vi "canDataSort.vi"() -> ()   [LabVIEW 2023] (continued)
  68\t00\t97\tCC\t00\t16\t39\t67\r\n      1542  18F120F0   00000004    8        2B\t75\t60\tB1\tB0\t01\tFF\tFF\r\n      1563  0CF101A7   00000004    8        68\t00\t97\tCC\t00\t16\t39\t68\r\n      1562  1FFFFFFF   00000004    8        00\t00\tFF\tFF\tFF\tFF\tFF\tFF\r\n      1552  1FFFFFFF   00000004    8        00\t00\tFF\tFF\tFF\tFF\tFF\tFF\r\n      1547  1FFFFFFF   00000004    8        00\t00\tFF\tFF\tFF\tFF\tFF\tFF\r\n      1546  18F121F0   00000004    8        09\t18\t00\t00\tFF\tFF\tB0\t01\r\n      1545  18F106A7   00000004    8        00\tF7\tFF\tFF\tFF\tFF\tFF\t8F\r\n      1545  0CF104A7   00000004    8        F0\t60\t22\tFC\tFF\tFF\tFF\t47\r\n      1544  0CF103A7   00000004    8        17\t1F\t08\t60\tB1\t1F\t08\t47\r\n      1544  0CF102A7   00000004    8        30\t75\tE0\t2E\t80\tFF\tFF\tFD\r\n      1543  0C3C4D4A   00000004    8        BE\tFF\tFF\t7F\t18\tFF\tFF\t47\r\n      1543  0CF101A7   00000004    8        68\t00\t97\tCC\t00\t16\t39\t67\r\n      1563  0CF102A7   00000004    8        30\t75\tE0\t2E\t80\tFF\tFF\tFD\r\n      1563  0CF101A7   00000004    8        68\t00\t97\tCC\t00\t16\t39\t68\r\n      1562  1FFFFFFF   00000004    8        00\t00\tFF\tFF\tFF\tFF\tFF\tFF\r\n      1552  1FFFFFFF   00000004    8        00\t00\tFF\tFF\tFF\tFF\tFF\tFF\r\n      1547  1FFFFFFF   00000004    8        00\t00\tFF\tFF\tFF\tFF\tFF\tFF\r\n      1546  18F121F0   00000004    8        09\t18\t00\t00\tFF\tFF\tB0\t01\r\n      1545  18F106A7   00000004    8        00\tF7\tFF\tFF\tFF\tFF\tFF\t8F\r\n      1545  0CF104A7   00000004    8        F0\t60\t22\tFC\tFF\tFF\tFF\t47\r\n      1544  0CF103A7   00000004    8        17\t1F\t08\t60\tB1\t1F\t08\t47\r\n      1544  0CF102A7   00000004    8        30\t75\tE0\t2E\t80\tFF\tFF\tFD\r\n      1543  0C3C4D4A   00000004    8        BE\tFF\tFF\t7F\t18\tFF\tFF\t47\r\n      1572  1FFFFFFF   00000004    8        00\t00\tFF\tFF\tFF\tFF\tFF\tFF\r\n      1563  0CF102A7   00000004    8        30\t75\tE0\t2E\t80\tFF\tFF\tFD\r\n      1563  0CF101A7   00000004    8        68\t00\t97\tCC\t00\t16\t39\t68\r\n      1562  1FFFFFFF   00000004    8        00\t00\tFF\tFF\tFF\tFF\tFF\tFF\r\n      1552  1FFFFFFF   00000004    8        00\t00\tFF\tFF\tFF\tFF\tFF\tFF\r\n      1547  1FFFFFFF   00000004    8        00\t00\tFF\tFF\tFF\tFF\tFF\tFF\r\n      1546  18F121F0   00000004    8        09\t18\t00\t00\tFF\tFF\tB0\t01\r\n      1545  18F106A7   00000004    8        00\tF7\tFF\tFF\tFF\tFF\tFF\t8F\r\n      1545  0CF104A7   00000004    8        F0\t60\t22\tFC\tFF\tFF\tFF\t47\r\n      1544  0CF103A7   00000004    8        17\t1F\t08\t60\tB1\t1F\t08\t47\r\n      1544  0CF102A7   00000004    8        30\t75\tE0\t2E\t80\tFF\tFF\tFD\r\n      1582  1FFFFFFF   00000004    8        00\t00\tFF\tFF\tFF\tFF\tFF\tFF\r\n      1572  1FFFFFFF   00000004    8        00\t00\tFF\tFF\tFF\tFF\tFF\tFF\r\n      1563  0CF102A7   00000004    8        30\t75\tE0\t2E\t80\tFF\tFF\tFD\r\n      1563  0CF101A7   00000004    8        68\t00\t97\tCC\t00\t16\t39\t68\r\n      1562  1FFFFFFF   00000004    8        00\t00\tFF\tFF\tFF\tFF\tFF\tFF\r\n      1552  1FFFFFFF   00000004    8        00\t00\tFF\tFF\tFF\tFF\tFF\tFF\r\n      1547  1FFFFFFF   00000004    8        00\t00\tFF\tFF\tFF\tFF\tFF\tFF\r\n      1546  18F121F0   00000004    8        09\t18\t00\t00\tFF\tFF\tB0\t01\r\n      1545  18F106A7   00000004    8        00\tF7\tFF\tFF\tFF\tFF\tFF\t8F\r\n      1545  0CF104A7   00000004    8        F0\t60\t22\tFC\tFF\tFF\tFF\t47\r\n      1544  0CF103A7   00000004    8        17\t1F\t08\t60\tB1\t1F\t08\t47\r\n      1583  0CF101A7   00000004    8        68\t00\t97\tCC\t00\t16\t39\t69\r\n      1582  1FFFFFFF   00000004    8        00\t00\tFF\tFF\tFF\tFF\tFF\tFF\r\n      1572  1FFFFFFF   00000004    8        00\t00\tFF\tFF\tFF\tFF\tFF\tFF\r\n      1563  0CF102A7   00000004    8        30\t75\tE0\t2E\t80\tFF\tFF\tFD\r\n      1563  0CF101A7   00000004    8        68\t00\t97\tCC\t00\t16\t39\t68\r\n      1562  1FFFFFFF   00000004    8        00\t00\tFF\tFF\tFF\tFF\tFF\tFF\r\n      1552  1FFFFFFF   00000004    8        00\t00\tFF\tFF\tFF\tFF\tFF\tFF\r\n      1547  1FFFFFFF   00000004    8        00\t00\tFF\tFF\tFF\tFF\tFF\tFF\r\n      1546  18F121F0   00000004    8        09\t18\t00\t00\tFF\tFF\tB0\t01\r\n      1545  18F106A7   00000004    8        00\tF7\tFF\tFF\tFF\tFF\tFF\t8F\r\n      1545  0CF104A7   00000004    8        F0\t60\t22\tFC\tFF\tFF\tFF\t47\r\n      1583  0CF102A7   00000004    8        30\t75\tE0\t2E\t80\tFF\tFF\tFD\r\n      1583  0CF101A7   00000004    8        68\t00\t97\tCC\t00\t16\t39\t69\r\n      1582  1FFFFFFF   00000004    8        00\t00\tFF\tFF\tFF\tFF\tFF\tFF\r\n      1572  1FFFFFFF   00000004    8        00\t00\tFF\tFF\tFF\tFF\tFF\tFF\r\n      1563  0CF102A7   00000004    8        30\t75\tE0\t2E\t80\tFF\tFF\tFD\r\n      1563  0CF101A7   00000004    8        68\t00\t97\tCC\t00\t16\t39\t68\r\n      1562  1FFFFFFF   00000004    8        00\t00\tFF\tFF\tFF\tFF\tFF\tFF\r\n      1552  1FFFFFFF   00000004    8        00\t00\tFF\tFF\tFF\tFF\tFF\tFF\r\n      1547  1FFFFFFF   00000004    8        00\t00\tFF\tFF\tFF\tFF\tFF\tFF\r\n      1546  18F121F0   00000004    8        09\t18\t00\t00\tFF\tFF\tB0\t01\r\n      1545  18F106A7   00000004    8        00\tF7\tFF\tFF\tFF\tFF\tFF\t8F\r\n      1592  1FFFFFFF   00000004    8        00\t00\tFF\tFF\tFF\tFF\tFF\tFF\r\n      1583  0CF102A7   00000004    8        30\t75\tE0\t2E\t80\tFF\tFF\tFD\r\n      1583  0CF101A7   00000004    8        68\t00\t97\tCC\t00\t16\t39\t69\r\n      1582  1FFFFFFF   00000004    8        00\t00\tFF\tFF\tFF\tFF\tFF\tFF\r\n      1572  1FFFFFFF   00000004    8        00\t00\tFF\tFF\tFF\tFF\tFF\tFF\r\n      1563  0CF102A7   00000004    8        30\t75\tE0\t2E\t80\tFF\tFF\tFD\r\n      1563  0CF101A7   00000004    8        68\t00\t97\tCC\t00\t16\t39\t68\r\n      1562  1FFFFFFF   00000004    8        00\t00\tFF\tFF\tFF\tFF\tFF\tFF\r\n      1552  1FFFFFFF   00000004    8        00\t00\tFF\tFF\tFF\tFF\tFF\tFF\r\n      1547  1FFFFFFF   00000004    8        00\t00\tFF\tFF\tFF\tFF\tFF\tFF\r\n      1546  18F121F0   00000004    8        09\t18\t00\t00\tFF\tFF\tB0\t01\r\n      1593  18F106A7   00000004    8        00\tF7\tFF\tFF\tFF\tFF\tFF\t90\r\n      1592  1FFFFFFF   00000004    8        00\t00\tFF\tFF\tFF\tFF\tFF\tFF\r\n      1583  0CF102A7   00000004    8        30\t75\tE0\t2E\t80\tFF\tFF\tFD\r\n      1583  0CF101A7   00000004    8        68\t00\t97\tCC\t00\t16\t39\t69\r\n      1582  1FFFFFFF   00000004    8        00\t00\tFF\tFF\tFF\tFF\tFF\tFF\r\n      1572  1FFFFFFF   00000004    8        00\t00\tFF\tFF\tFF\tFF\tFF\tFF\r\n      1563  0CF102A7   00000004    8        30\t75\tE0\t2E\t80\tFF\tFF\tFD\r\n      1563  0CF101A7   00000004    8        68\t00\t97\tCC\t00\t16\t39\t68\r\n      1562  1FFFFFFF   00000004    8        00\t00\tFF\tFF\tFF\tFF\tFF\tFF\r\n      1552  1FFFFFFF   00000004    8        00\t00\tFF\tFF\tFF\tFF\tFF\tFF\r\n      1547  1FFFFFFF   00000004    8        00\t00\tFF\tFF\tFF\tFF\tFF\tFF\r\n      1602  1FFFFFFF   00000004    8        00\t00\tFF\tFF\tFF\tFF\tFF\tFF\r\n      1593  18F106A7   00000004    8        00\tF7\tFF\tFF\tFF\tFF\tFF\t90\r\n      1592  1FFFFFFF   00000004    8        00\t00\tFF\tFF\tFF\tFF\tFF\tFF\r\n      1583  0CF102A7   00000004    8        30\t75\tE0\t2E\t80\tFF\tFF\tFD\r\n      1583  0CF101A7   00000004    8        68\t00\t97\tCC\t00\t16\t39\t69\r\n      1582  1FFFFFFF   00000004    8        00\t00\tFF\tFF\tFF\tFF\tFF\tFF\r\n      1572  1FFFFFFF   00000004    8        00\t00\tFF\tFF\tFF\tFF\tFF\tFF\r\n      1563  0CF102A7   00000004    8        30\t75\tE0\t2E\t80\tFF\tFF\tFD\r\n      1563  0CF101A7   00000004    8        68\t00\t97\tCC\t00\t16\t39\t68\r\n      1562  1FFFFFFF   00000004    8        00\t00\tFF\tFF\tFF\tFF\tFF\tFF\r\n      1552  1FFFFFFF   00000004    8        00\t00\tFF\tFF\tFF\tFF\tFF\tFF\r\n      1603  0CF101A7   00000004    8        68\t00\t97\tCC\t00\t16\t39\t6A\r\n      1602  1FFFFFFF   00000004    8        00\t00\tFF\tFF\tFF\tFF\tFF\tFF\r\n      1593  18F106A7   00000004    8        00\tF7\tFF\tFF\tFF\tFF\tFF\t90\r\n      1592  1FFFFFFF   00000004    8        00\t00\tFF\tFF\tFF\tFF\tFF\tFF\r\n      1583  0CF102A7   00000004    8        30\t75\tE0\t2E\t80\tFF\tFF\tFD\r\n      1583  0CF101A7   00000004    8        68\t00\t97\tCC\t00\t16\t39\t69\r\n      1582  1FFFFFFF   00000004    8        00\t00\tFF\tFF\tFF\tFF\tFF\tFF\r\n      1572  1FFFFFFF   00000004    8        00\t00\tFF\tFF\tFF\tFF\tFF\tFF\r\n      1563  0CF102A7   00000004    8        30\t75\tE0\t2E\t80\tFF\tFF\tFD\r\n      1563  0CF101A7   00000004    8        68\t00\t97\tCC\t00\t16\t39\t68\r\n      1562  1FFFFFFF   00000004    8        00\t00\tFF\tFF\tFF\tFF\tFF\tFF\r\n      1603  0CF102A7   00000004    8        30\t75\tE0\t2E\t80\tFF\tFF\tFD\r\n      1603  0CF101A7   00000004    8        68\t00\t97\tCC\t00\t16\t39\t6A\r\n      1602  1FFFFFFF   00000004    8        00\t00\tFF\tFF\tFF\tFF\tFF\tFF\r\n      1593  18F106A7   00000004    8        00\tF7\tFF\tFF\tFF\tFF\tFF\t90\r\n      1592  1FFFFFFF   00000004    8        00\t00\tFF\tFF\tFF\tFF\tFF\tFF\r\n      1583  0CF102A7   00000004    8        30\t75\tE0\t2E\t80\tFF\tFF\tFD\r\n      1583  0CF101A7   00000004    8        68\t00\t97\tCC\t00\t16\t39\t69\r\n      1582  1FFFFFFF   00000004    8        00\t00\tFF\tFF\tFF\tFF\tFF\tFF\r\n      1572  1FFFFFFF   00000004    8        00\t00\tFF\tFF\tFF\tFF\tFF\tFF\r\n      1563  0CF102A7   00000004    8        30\t75\tE0\t2E\t80\tFF\tFF\tFD\r\n      1563  0CF101A7   00000004    8        68\t00\t97\tCC\t00\t16\t39\t68\r\n      1612  1FFFFFFF   00000004    8        00\t00\tFF\tFF\tFF\tFF\tFF\tFF\r\n      1603  0CF102A7   00000004    8        30\t75\tE0\t2E\t80\tFF\tFF\tFD\r\n      1603  0CF101A7   00000004    8        68\t00\t97\tCC\t00\t16\t39\t6A\r\n      1602  1FFFFFFF   00000004    8        00\t00\tFF\tFF\tFF\tFF\tFF\tFF\r\n      1593  18F106A7   00000004    8        00\tF7\tFF\tFF\tFF\tFF\tFF\t90\r\n      1592  1FFFFFFF   00000004    8        00\t00\tFF\tFF\tFF\tFF\tFF\tFF\r\n      1583  0CF102A7   00000004    8        30\t75\tE0\t2E\t80\tFF\tFF\tFD\r\n      1583  0CF101A7   00000004    8        68\t00\t97\tCC\t00\t16\t39\t69\r\n      1582  1FFFFFFF   00000004    8        00\t00\tFF\tFF\tFF\tFF\tFF\tFF\r\n      1572  1FFFFFFF   00000004    8        00\t00\tFF\tFF\tFF\tFF\tFF\tFF\r\n      1563  0CF102A7   00000004    8        30\t75\tE0\t2E\t80\tFF\tFF\tFD\r\n      1622  1FFFFFFF   00000004    8        00\t00\tFF\tFF\tFF\tFF\tFF\tFF\r\n      1612  1FFFFFFF   00000004    8        00\t00\tFF\tFF\tFF\tFF\tFF\tFF\r\n      1603  0CF102A7   00000004    8        30\t75\tE0\t2E\t80\tFF\tFF\tFD\r\n      1603  0CF101A7   00000004    8        68\t00\t97\tCC\t00\t16\t39\t6A\r\n      1602  1FFFFFFF   00000004    8        00\t00\tFF\tFF\tFF\tFF\tFF\tFF\r\n      1593  18F106A7   00000004    8        00\tF7\tFF\tFF\tFF\tFF\tFF\t90\r\n      1592  1FFFFFFF   00000004    8        00\t00\tFF\tFF\tFF\tFF\tFF\tFF\r\n      1583  0CF102A7   00000004    8        30\t75\tE0\t2E\t80\tFF\tFF\tFD\r\n      1583  0CF101A7   00000004    8        68\t00\t97\tCC\t00\t16\t39\t69\r\n      1582  1FFFFFFF   00000004    8        00\t00\tFF\tFF\tFF\tFF\tFF\tFF\r\n      1572  1FFFFFFF   00000004    8        00\t00\tFF\tFF\tFF\tFF\tFF\tFF\r\n      1623  0CF101A7   00000004    8        68\t00\t97\tCC\t00\t16\t39\t6B\r\n      1622  1FFFFFFF   00000004    8        00\t00\tFF\tFF\tFF\tFF\tFF\tFF\r\n      1612  1FFFFFFF   00000004    8        00\t00\tFF\tFF\tFF\tFF\tFF\tFF\r\n      1603  0CF102A7   00000004    8        30\t75\tE0\t2E\t80\tFF\tFF\tFD\r\n      1603  0CF101A7   00000004    8        68\t00\t97\tCC\t00\t16\t39\t6A\r\n      1602  1FFFFFFF   00000004    8        00\t00\tFF\tFF\tFF\tFF\tFF\tFF\r\n      1593  18F106A7   00000004    8        00\tF7\tFF\tFF\tFF\tFF\tFF\t90\r\n      1592  1FFFFFFF   00000004    8        00\t00\tFF\tFF\tFF\tFF\tFF\tFF\r\n      1583  0CF102A7   00000004    8        30\t75\tE0\t2E\t80\tFF\tFF\tFD\r\n      1583  0CF101A7   00000004    8        68\t00\t97\tCC\t00\t16\t39\t69\r\n      1582  1FFFFFFF   00000004    8        00\t00\tFF\tFF\tFF\tFF\tFF\tFF\r\n      1623  0CF102A7   00000004    8        30\t75\tE0\t2E\t80\tFF\tFF\tFD\r\n      1623  0CF101A7   00000004    8        68\t00\t97\tCC\t00\t16\t39\t6B\r\n      1622  1FFFFFFF   00000004    8        00\t00\tFF\tFF\tFF\tFF\tFF\tFF\r\n      1612  1FFFFFFF   00000004    8        00\t00\tFF\tFF\tFF\tFF\tFF\tFF\r\n      1603  0CF102A7   00000004    8        30\t75\tE0\t2E\t80\tFF\tFF\tFD\r\n      1603  0CF101A7   00000004    8        68\t00\t97\tCC\t00\t16\t39\t6A\r\n      1602  1FFFFFFF   00000004    8        00\t00\tFF\tFF\tFF\tFF\tFF\tFF\r\n      1593  18F106A7   00000004    8        00\tF7\tFF\tFF\tFF\tFF\tFF\t90\r\n      1592  1FFFFFFF   00000004    8        00\t00\tFF\tFF\tFF\tFF\tFF\tFF\r\n      1583  0CF102A7   00000004    8        30\t75\tE0\t2E\t80\tFF\tFF\tFD\r\n      1583  0CF101A7   00000004    8        68\t00\t97\tCC\t00\t16\t39\t69\r\n      1632  1FFFFFFF   00000004    8        00\t00\tFF\tFF\tFF\tFF\tFF\tFF\r\n      1623  0CF102A7   00000004    8        30\t75\tE0\t2E\t80\tFF\tFF\tFD\r\n      1623  0CF101A7   00000004    8        68\t00\t97\tCC\t00\t16\t39\t6B\r\n      1622  1FFFFFFF   00000004    8        00\t00\tFF\tFF\tFF\tFF\tFF\tFF\r\n      1612  1FFFFFFF   00000004    8        00\t00\tFF\tFF\tFF\tFF\tFF\tFF\r\n      1603  0CF102A7   00000004    8        30\t75\tE0\t2E\t80\tFF\tFF\tFD\r\n      1603  0CF101A7   00000004    8        68\t00\t97\tCC\t00\t16\t39\t6A\r\n      1602  1FFFFFFF   00000004    8        00\t00\tFF\tFF\tFF\tFF\tFF\tFF\r\n      1593  18F106A7   00000004    8        00\tF7\tFF\tFF\tFF\tFF\tFF\t90\r\n      1592  1FFFFFFF   00000004    8        00\t00\tFF\tFF\tFF\tFF\tFF\tFF\r\n      1583  0CF102A7   00000004    8        30\t75\tE0\t2E\t80\tFF\tFF\tFD\r\n      1642  18F11FF0   00000004    8        FF\t3F\t90\t68\t88\t1B\t10\t8C\r\n      1632  1FFFFFFF   00000004    8        00\t00\tFF\tFF\tFF\tFF\tFF\tFF\r\n      1623  0CF102A7   00000004    8        30\t75\tE0\t2E\t80\tFF\tFF\tFD\r\n      1623  0CF101A7   00000004    8        68\t00\t97\tCC\t00\t16\t39\t6B\r\n      1622  1FFFFFFF   00000004    8        00\t00\tFF\tFF\tFF\tFF\tFF\tFF\r\n      1612  1FFFFFFF   00000004    8        00\t00\tFF\tFF\tFF\tFF\tFF\tFF\r\n      1603  0CF102A7   00000004    8        30\t75\tE0\t2E\t80\tFF\tFF\tFD\r\n      1603  0CF101A7   00000004    8        68\t00\t97\tCC\t00\t16\t39\t6A\r\n      1602  1FFFFFFF   00000004    8        00\t00\tFF\tFF\tFF\tFF\tFF\tFF\r\n      1593  18F106A7   00000004    8        00\tF7\tFF\tFF\tFF\tFF\tFF\t90\r\n      1592  1FFFFFFF   00000004    8        00\t00\tFF\tFF\tFF\tFF\tFF\tFF\r\n      1643  0CF101A7   00000004    8        68\t00\t97\tCC\t00\t16\t39\t6C\r\n      1642  18F11FF0   00000004    8        FF\t3F\t90\t68\t88\t1B\t10\t8C\r\n      1632  1FFFFFFF   00000004    8        00\t00\tFF\tFF\tFF\tFF\tFF\tFF\r\n      1623  0CF102A7   00000004    8        30\t75\tE0\t2E\t80\tFF\tFF\tFD\r\n      1623  0CF101A7   00000004    8        68\t00\t97\tCC\t00\t16\t39\t6B\r\n      1622  1FFFFFFF   00000004    8        00\t00\tFF\tFF\tFF\tFF\tFF\tFF\r\n      1612  1FFFFFFF   00000004    8        00\t00\tFF\tFF\tFF\tFF\tFF\tFF\r\n      1603  0CF102A7   00000004    8        30\t75\tE0\t2E\t80\tFF\tFF\tFD\r\n      1603  0CF101A7   00000004    8        68\t00\t97\tCC\t00\t16\t39\t6A\r\n      1602  1FFFFFFF   00000004    8        00\t00\tFF\tFF\tFF\tFF\tFF\tFF\r\n      1593  18F106A7   00000004    8        00\tF7\tFF\tFF\tFF\tFF\tFF\t90\r\n      1643  0CF102A7   00000004    8        30\t75\tE0\t2E\t80\tFF\tFF\tFD\r\n      1643  0CF101A7   00000004    8        68\t00\t97\tCC\t00\t16\t39\t6C\r\n      1642  18F11FF0   00000004    8        FF\t3F\t90\t68\t88\t1B\t10\t8C\r\n      1632  1FFFFFFF   00000004    8        00\t00\tFF\tFF\tFF\tFF\tFF\tFF\r\n      1623  0CF102A7   00000004    8        30\t75\tE0\t2E\t80\tFF\tFF\tFD\r\n      1623  0CF101A7   00000004    8        68\t00\t97\tCC\t00\t16\t39\t6B\r\n      1622  1FFFFFFF   00000004    8        00\t00\tFF\tFF\tFF\tFF\tFF\tFF\r\n      1612  1FFFFFFF   00000004    8        00\t00\tFF\tFF\tFF\tFF\tFF\tFF\r\n      1603  0CF102A7   00000004    8        30\t75\tE0\t2E\t80\tFF\tFF\tFD\r\n      1603  0CF101A7   00000004    8        68\t00\t97\tCC\t00\t16\t39\t6A\r\n      1602  1FFFFFFF   00000004    8        00\t00\tFF\tFF\tFF\tFF\tFF\tFF\r\n      1644  0C3C4D4A   00000004    8        BE\tFF\tFF\t7F\t18\tFF\tFF\t48\r\n      1643  0CF102A7   00000004    8        30\t75\tE0\t2E\t80\tFF\tFF\tFD\r\n      1643  0CF101A7   00000004    8        68\t00\t97\tCC\t00\t16\t39\t6C\r\n      1642  18F11FF0   00000004    8        FF\t3F\t90\t68\t88\t1B\t10\t8C\r\n      1632  1FFFFFFF   00000004    8        00\t00\tFF\tFF\tFF\tFF\tFF\tFF\r\n      1623  0CF102A7   00000004    8        30\t75\tE0\t2E\t80\tFF\tFF\tFD\r\n      1623  0CF101A7   00000004    8        68\t00\t97\tCC\t00\t16\t39\t6B\r\n      1622  1FFFFFFF   00000004    8        00\t00\tFF\tFF\tFF\tFF\tFF\tFF\r\n      1612  1FFFFFFF   00000004    8        00\t00\tFF\tFF\tFF\tFF\tFF\tFF\r\n      1603  0CF102A7   00000004    8        30\t75\tE0\t2E\t80\tFF\tFF\tFD\r\n      1603  0CF101A7   00000004    8        68\t00\t97\tCC\t00\t16\t39\t6A\r\n      1644  0CF103A7   00000004    8        17\t1F\t08\t60\tB1\t1F\t08\t48\r\n      1644  0C3C4D4A   00000004    8        BE\tFF\tFF\t7F\t18\tFF\tFF\t48\r\n      1643  0CF102A7   00000004    8        30\t75\tE0\t2E\t80\tFF\tFF\tFD\r\n      1643  0CF101A7   00000004    8        68\t00\t97\tCC\t00\t16\t39\t6C\r\n      1642  18F11FF0   00000004    8        FF\t3F\t90\t68\t88\t1B\t10\t8C\r\n      1632  1FFFFFFF   00000004    8        00\t00\tFF\tFF\tFF\tFF\tFF\tFF\r\n      1623  0CF102A7   00000004    8        30\t75\tE0\t2E\t80\tFF\tFF\tFD\r\n      1623  0CF101A7   00000004    8        68\t00\t97\tCC\t00\t16\t39\t6B\r\n      1622  1FFFFFFF   00000004    8        00\t00\tFF\tFF\tFF\tFF\tFF\tFF\r\n      1612  1FFFFFFF   00000004    8        00\t00\tFF\tFF\tFF\tFF\tFF\tFF\r\n      1603  0CF102A7   00000004    8        30\t75\tE0\t2E\t80\tFF\tFF\tFD\r\n      1645  0CF104A7   00000004    8        F0\t60\t22\tFC\tFF\tFF\tFF\t48\r\n      1644  0CF103A7   00000004    8        17\t1F\t08\t60\tB1\t1F\t08\t48\r\n      1644  0C3C4D4A   00000004    8        BE\tFF\tFF\t7F\t18\tFF\tFF\t48\r\n      1643  0CF102A7   00000004    8        30\t75\tE0\t2E\t80\tFF\tFF\tFD\r\n      1643  0CF101A7   00000004    8        68\t00\t97\tCC\t00\t16\t39\t6C\r\n      1642  18F11FF0   00000004    8        FF\t3F\t90\t68\t88\t1B\t10\t8C\r\n      1632  1FFFFFFF   00000004    8        00\t00\tFF\tFF\tFF\tFF\tFF\tFF\r\n      1623  0CF102A7   00000004    8        30\t75\tE0\t2E\t80\tFF\tFF\tFD\r\n      1623  0CF101A7   00000004    8        68\t00\t97\tCC\t00\t16\t39\t6B\r\n      1622  1FFFFFFF   00000004    8        00\t00\tFF\tFF\tFF\tFF\tFF\tFF\r\n      1612  1FFFFFFF   00000004    8        00\t00\tFF\tFF\tFF\tFF\tFF\tFF\r\n      1645  0CF105A7   00000004    8        94\t11\t00\t55\tFF\tFF\tFF\t20\r\n      1645  0CF104A7   00000004    8        F0\t60\t22\tFC\tFF\tFF\tFF\t48\r\n      1644  0CF103A7   00000004    8        17\t1F\t08\t60\tB1\t1F\t08\t48\r\n      1644  0C3C4D4A   00000004    8        BE\tFF\tFF\t7F\t18\tFF\tFF\t48\r\n      1643  0CF102A7   00000004    8        30\t75\tE0\t2E\t80\tFF\tFF\tFD\r\n      1643  0CF101A7   00000004    8        68\t00\t97\tCC\t00\t16\t39\t6C\r\n      1642  18F11FF0   00000004    8        FF\t3F\t90\t68\t88\t1B\t10\t8C\r\n      1632  1FFFFFFF   00000004    8        00\t00\tFF\tFF\tFF\tFF\tFF\tFF\r\n      1623  0CF102A7   00000004    8        30\t75\tE0\t2E\t80\tFF\tFF\tFD\r\n      1623  0CF101A7   00000004    8        68\t00\t97\tCC\t00\t16\t39\t6B\r\n      1622  1FFFFFFF   00000004    8        00\t00\tFF\tFF\tFF\tFF\tFF\tFF\r\n      1646  18F106A7   00000004    8        00\tF7\tFF\tFF\tFF\tFF\tFF\t91\r\n      1645  0CF105A7   00000004    8        94\t11\t00\t55\tFF\tFF\tFF\t20\r\n      1645  0CF104A7   00000004    8        F0\t60\t22\tFC\tFF\tFF\tFF\t48\r\n      1644  0CF103A7   00000004    8        17\t1F\t08\t60\tB1\t1F\t08\t48\r\n      1644  0C3C4D4A   00000004    8        BE\tFF\tFF\t7F\t18\tFF\tFF\t48\r\n      1643  0CF102A7   00000004    8        30\t75\tE0\t2E\t80\tFF\tFF\tFD\r\n      1643  0CF101A7   00000004    8        68\t00\t97\tCC\t00\t16\t39\t6C\r\n      1642  18F11FF0   00000004    8        FF\t3F\t90\t68\t88\t1B\t10\t8C\r\n      1632  1FFFFFFF   00000004    8        00\t00\tFF\tFF\tFF\tFF\tFF\tFF\r\n      1623  0CF102A7   00000004    8        30\t75\tE0\t2E\t80\tFF\tFF\tFD\r\n      1623  0CF101A7   00000004    8        68\t00\t97\tCC\t00\t16\t39\t6B\r\n      1647  18F108A7   00000004    8        F0\t00\t00\tFF\tFF\tFF\tFF\t41\r\n      1646  18F106A7   00000004    8        00\tF7\tFF\tFF\tFF\tFF\tFF\t91\r\n      1645  0CF105A7   00000004    8        94\t11\t00\t55\tFF\tFF\tFF\t20\r\n      1645  0CF104A7   00000004    8        F0\t60\t22\tFC\tFF\tFF\tFF\t48\r\n      1644  0CF103A7   00000004    8        17\t1F\t08\t60\tB1\t1F\t08\t48\r\n      1644  0C3C4D4A   00000004    8        BE\tFF\tFF\t7F\t18\tFF\tFF\t48\r\n      1643  0CF102A7   00000004    8        30\t75\tE0\t2E\t80\tFF\tFF\tFD\r\n      1643  0CF101A7   00000004    8        68\t00\t97\tCC\t00\t16\t39\t6C\r\n      1642  18F11FF0   00000004    8        FF\t3F\t90\t68\t88\t1B\t10\t8C\r\n      1632  1FFFFFFF   00000004    8        00\t00\tFF\tFF\tFF\tFF\tFF\tFF\r\n      1623  0CF102A7   00000004    8        30\t75\tE0\t2E\t80\tFF\tFF\tFD\r\n      1647  18F120F0   00000004    8        2B\t75\t60\tB1\tB0\t01\tFF\tFF\r\n      1647  18F108A7   00000004    8        F0\t00\t00\tFF\tFF\tFF\tFF\t41\r\n      1646  18F106A7   00000004    8        00\tF7\tFF\tFF\tFF\tFF\tFF\t91\r\n      1645  0CF105A7   00000004    8        94\t11\t00\t55\tFF\tFF\tFF\t20\r\n      1645  0CF104A7   00000004    8        F0\t60\t22\tFC\tFF\tFF\tFF\t48\r\n      1644  0CF103A7   00000004    8        17\t1F\t08\t60\tB1\t1F\t08\t48\r\n      1644  0C3C4D4A   00000004    8        BE\tFF\tFF\t7F\t18\tFF\tFF\t48\r\n      1643  0CF102A7   00000004    8        30\t75\tE0\t2E\t80\tFF\tFF\tFD\r\n      1643  0CF101A7   00000004    8        68\t00\t97\tCC\t00\t16\t39\t6C\r\n      1642  18F11FF0   00000004    8        FF\t3F\t90\t68\t88\t1B\t10\t8C\r\n      1632  1FFFFFFF   00000004    8        00\t00\tFF\tFF\tFF\tFF\tFF\tFF\r\n      1648  18F121F0   00000004    8        09\t18\t00\t00\tFF\tFF\tB0\t01\r\n      1647  18F120F0   00000004    8        2B\t75\t60\tB1\tB0\t01\tFF\tFF\r\n      1647  18F108A7   00000004    8        F0\t00\t00\tFF\tFF\tFF\tFF\t41\r\n      1646  18F106A7   00000004    8        00\tF7\tFF\tFF\tFF\tFF\tFF\t91\r\n      1645  0CF105A7   00000004    8        94\t11\t00\t55\tFF\tFF\tFF\t20\r\n      1645  0CF104A7   00000004    8        F0\t60\t22\tFC\tFF\tFF\tFF\t48\r\n      1644  0CF103A7   00000004    8        17\t1F\t08\t60\tB1\t1F\t08\t48\r\n      1644  0C3C4D4A   00000004    8        BE\tFF\tFF\t7F\t18\tFF\tFF\t48\r\n      1643  0CF102A7   00000004    8        30\t75\tE0\t2E\t80\tFF\tFF\tFD\r\n      1643  0CF101A7   00000004    8        68\t00\t97\tCC\t00\t16\t39\t6C\r\n      1642  18F11FF0   00000004    8        FF\t3F\t90\t68\t88\t1B\t10\t8C\r\n      1648  18FB01A7   00000004    8        FF\t1F\tFF\tFF\tFF\tFF\tFF\tFF\r\n      1648  18F121F0   00000004    8        09\t18\t00\t00\tFF\tFF\tB0\t01\r\n      1647  18F120F0   00000004    8        2B\t75\t60\tB1\tB0\t01\tFF\tFF\r\n      1647  18F108A7   00000004    8        F0\t00\t00\tFF\tFF\tFF\tFF\t41\r\n      1646  18F106A7   00000004    8        00\tF7\tFF\tFF\tFF\tFF\tFF\t91\r\n      1645  0CF105A7   00000004    8        94\t11\t00\t55\tFF\tFF\tFF\t20\r\n      1645  0CF104A7   00000004    8        F0\t60\t22\tFC\tFF\tFF\tFF\t48\r\n      1644  0CF103A7   00000004    8        17\t1F\t08\t60\tB1\t1F\t08\t48\r\n      1644  0C3C4D4A   00000004    8        BE\tFF\tFF\t7F\t18\tFF\tFF\t48\r\n      1643  0CF102A7   00000004    8        30\t75\tE0\t2E\t80\tFF\tFF\tFD\r\n      1643  0CF101A7   00000004    8        68\t00\t97\tCC\t00\t16\t39\t6C\r\n      1649  18FEF117   00000004    8        F7\t97\tCC\tCF\tFF\tFF\tFF\tFF\r\n      1648  18FB01A7   00000004    8        FF\t1F\tFF\tFF\tFF\tFF\tFF\tFF\r\n      1648  18F121F0   00000004    8        09\t18\t00\t00\tFF\tFF\tB0\t01\r\n      1647  18F120F0   00000004    8        2B\t75\t60\tB1\tB0\t01\tFF\tFF\r\n      1647  18F108A7   00000004    8        F0\t00\t00\tFF\tFF\tFF\tFF\t41\r\n      1646  18F106A7   00000004    8        00\tF7\tFF\tFF\tFF\tFF\tFF\t91\r\n      1645  0CF105A7   00000004    8        94\t11\t00\t55\tFF\tFF\tFF\t20\r\n      1645  0CF104A7   00000004    8        F0\t60\t22\tFC\tFF\tFF\tFF\t48\r\n      1644  0CF103A7   00000004    8        17\t1F\t08\t60\tB1\t1F\t08\t48\r\n      1644  0C3C4D4A   00000004    8        BE\tFF\tFF\t7F\t18\tFF\tFF\t48\r\n      1643  0CF102A7   00000004    8        30\t75\tE0\t2E\t80\tFF\tFF\tFD\r\n      1649  1FFFFFFF   00000004    8        00\t00\tFF\tFF\tFF\tFF\tFF\tFF\r\n      1649  18FEF117   00000004    8        F7\t97\tCC\tCF\tFF\tFF\tFF\tFF\r\n      1648  18FB01A7   00000004    8        FF\t1F\tFF\tFF\tFF\tFF\tFF\tFF\r\n      1648  18F121F0   00000004    8        09\t18\t00\t00\tFF\tFF\tB0\t01\r\n      1647  18F120F0   00000004    8        2B\t75\t60\tB1\tB0\t01\tFF\tFF\r\n      1647  18F108A7   00000004    8        F0\t00\t00\tFF\tFF\tFF\tFF\t41\r\n      1646  18F106A7   00000004    8        00\tF7\tFF\tFF\tFF\tFF\tFF\t91\r\n      1645  0CF105A7   00000004    8        94\t11\t00\t55\tFF\tFF\tFF\t20\r\n      1645  0CF104A7   00000004    8        F0\t60\t22\tFC\tFF\tFF\tFF\t48\r\n      1644  0CF103A7   00000004    8        17\t1F\t08\t60\tB1\t1F\t08\t48\r\n      1644  0C3C4D4A   00000004    8        BE\tFF\tFF\t7F\t18\tFF\tFF\t48\r\n      1652  1FFFFFFF   00000004    8        00\t20\tFF\tFF\tFF\tFF\tFF\tFF\r\n      1649  1FFFFFFF   00000004    8        00\t00\tFF\tFF\tFF\tFF\tFF\tFF\r\n      1649  18FEF117   00000004    8        F7\t97\tCC\tCF\tFF\tFF\tFF\tFF\r\n      1648  18FB01A7   00000004    8        FF\t1F\tFF\tFF\tFF\tFF\tFF\tFF\r\n      1648  18F121F0   00000004    8        09\t18\t00\t00\tFF\tFF\tB0\t01\r\n      1647  18F120F0   00000004    8        2B\t75\t60\tB1\tB0\t01\tFF\tFF\r\n      1647  18F108A7   00000004    8        F0\t00\t00\tFF\tFF\tFF\tFF\t41\r\n      1646  18F106A7   00000004    8        00\tF7\tFF\tFF\tFF\tFF\tFF\t91\r\n      1645  0CF105A7   00000004    8        94\t11\t00\t55\tFF\tFF\tFF\t20\r\n      1645  0CF104A7   00000004    8        F0\t60\t22\tFC\tFF\tFF\tFF\t48\r\n      1644  0CF103A7   00000004    8        17\t1F\t08\t60\tB1\t1F\t08\t48\r\n      1662  1FFFFFFF   00000004    8        00\t20\tFF\tFF\tFF\tFF\tFF\tFF\r\n      1652  1FFFFFFF   00000004    8        00\t20\tFF\tFF\tFF\tFF\tFF\tFF\r\n      1649  1FFFFFFF   00000004    8        00\t00\tFF\tFF\tFF\tFF\tFF\tFF\r\n      1649  18FEF117   00000004    8        F7\t97\tCC\tCF\tFF\tFF\tFF\tFF\r\n      1648  18FB01A7   00000004    8        FF\t1F\tFF\tFF\tFF\tFF\tFF\tFF\r\n      1648  18F121F0   00000004    8        09\t18\t00\t00\tFF\tFF\tB0\t01\r\n      1647  18F120F0   00000004    8        2B\t75\t60\tB1\tB0\t01\tFF\tFF\r\n      1647  18F108A7   00000004    8        F0\t00\t00\tFF\tFF\tFF\tFF\t41\r\n      1646  18F106A7   00000004    8        00\tF7\tFF\tFF\tFF\tFF\tFF\t91\r\n      1645  0CF105A7   00000004    8        94\t11\t00\t55\tFF\tFF\tFF\t20\r\n      1645  0CF104A7   00000004    8        F0\t60\t22\tFC\tFF\tFF\tFF\t48\r\n      1663  0CF101A7   00000004    8        68\t00\t97\tCC\t00\t16\t39\t6D\r\n      1662  1FFFFFFF   00000004    8        00\t20\tFF\tFF\tFF\tFF\tFF\tFF\r\n      1652  1FFFFFFF   00000004    8        00\t20\tFF\tFF\tFF\tFF\tFF\tFF\r\n      1649  1FFFFFFF   00000004    8        00\t00\tFF\tFF\tFF\tFF\tFF\tFF\r\n      1649  18FEF117   00000004    8        F7\t97\tCC\tCF\tFF\tFF\tFF\tFF\r\n      1648  18FB01A7   00000004    8        FF\t1F\tFF\tFF\tFF\tFF\tFF\tFF\r\n      1648  18F121F0   00000004    8        09\t18\t00\t00\tFF\tFF\tB0\t01\r\n      1647  18F120F0   00000004    8        2B\t75\t60\tB1\tB0\t01\tFF\tFF\r\n      1647  18F108A7   00000004    8        F0\t00\t00\tFF\tFF\tFF\tFF\t41\r\n      1646  18F106A7   00000004    8        00\tF7\tFF\tFF\tFF\tFF\tFF\t91\r\n      1645  0CF105A7   00000004    8        94\t11\t00\t55\tFF\tFF\tFF\t20\r\n      1663  0CF102A7   00000004    8        30\t75\tE0\t2E\t80\tFF\tFF\tFD\r\n      1663  0CF101A7   00000004    8        68\t00\t97\tCC\t00\t16\t39\t6D\r\n      1662  1FFFFFFF   00000004    8        00\t20\tFF\tFF\tFF\tFF\tFF\tFF\r\n      1652  1FFFFFFF   00000004    8        00\t20\tFF\tFF\tFF\tFF\tFF\tFF\r\n      1649  1FFFFFFF   00000004    8        00\t00\tFF\tFF\tFF\tFF\tFF\tFF\r\n      1649  18FEF117   00000004    8        F7\t97\tCC\tCF\tFF\tFF\tFF\tFF\r\n      1648  18FB01A7   00000004    8        FF\t1F\tFF\tFF\tFF\tFF\tFF\tFF\r\n      1648  18F121F0   00000004    8        09\t18\t00\t00\tFF\tFF\tB0\t01\r\n      1647  18F120F0   00000004    8        2B\t75\t60\tB1\tB0\t01\tFF\tFF\r\n      1647  18F108A7   00000004    8        F0\t00\t00\tFF\tFF\tFF\tFF\t41\r\n      1646  18F106A7   00000004    8        00\tF7\tFF\tFF\tFF\tFF\tFF\t91\r\n      1672  1FFFFFFF   00000004    8        00\t00\tFF\tFF\tFF\tFF\tFF\tFF\r\n      1663  0CF102A7   00000004    8        30\t75\tE0\t2E\t80\tFF\tFF\tFD\r\n      1663  0CF101A7   00000004    8        68\t00\t97\tCC\t00\t16\t39\t6D\r\n      1662  1FFFFFFF   00000004    8        00\t20\tFF\tFF\tFF\tFF\tFF\tFF\r\n      1652  1FFFFFFF   00000004    8        00\t20\tFF\tFF\tFF\tFF\tFF\tFF\r\n      1649  1FFFFFFF   00000004    8        00\t00\tFF\tFF\tFF\tFF\tFF\tFF\r\n      1649  18FEF117   00000004    8        F7\t97\tCC\tCF\tFF\tFF\tFF\tFF\r\n      1648  18FB01A7   00000004    8        FF\t1F\tFF\tFF\tFF\tFF\tFF\tFF\r\n      1648  18F121F0   00000004    8        09\t18\t00\t00\tFF\tFF\tB0\t01\r\n      1647  18F120F0   00000004    8        2B\t75\t60\tB1\tB0\t01\tFF\tFF\r\n      1647  18F108A7   00000004    8        F0\t00\t00\tFF\tFF\tFF\tFF\t41\r\n      1682  1FFFFFFF   00000004    8        00\t00\tFF\tFF\tFF\tFF\tFF\tFF\r\n      1672  1FFFFFFF   00000004    8        00\t00\tFF\tFF\tFF\tFF\tFF\tFF\r\n      1663  0CF102A7   00000004    8        30\t75\tE0\t2E\t80\tFF\tFF\tFD\r\n      1663  0CF101A7   00000004    8        68\t00\t97\tCC\t00\t16\t39\t6D\r\n      1662  1FFFFFFF   00000004    8        00\t20\tFF\tFF\tFF\tFF\tFF\tFF\r\n      1652  1FFFFFFF   00000004    8        00\t20\tFF\tFF\tFF\tFF\tFF\tFF\r\n      1649  1FFFFFFF   00000004    8        00\t00\tFF\tFF\tFF\tFF\tFF\tFF\r\n      1649  18FEF117   00000004    8        F7\t97\tCC\tCF\tFF\tFF\tFF\tFF\r\n      1648  18FB01A7   00000004    8        FF\t1F\tFF\tFF\tFF\tFF\tFF\tFF\r\n      1648  18F121F0   00000004    8        09\t18\t00\t00\tFF\tFF\tB0\t01\r\n      1647  18F120F0   00000004    8        2B\t75\t60\tB1\tB0\t01\tFF\tFF\r\n      1683  0CF101A7   00000004    8        68\t00\t97\tCC\t00\t16\t39\t6E\r\n      1682  1FFFFFFF   00000004    8        00\t00\tFF\tFF\tFF\tFF\tFF\tFF\r\n      1672  1FFFFFFF   00000004    8        00\t00\tFF\tFF\tFF\tFF\tFF\tFF\r\n      1663  0CF102A7   00000004    8        30\t75\tE0\t2E\t80\tFF\tFF\tFD\r\n      1663  0CF101A7   00000004    8        68\t00\t97\tCC\t00\t16\t39\t6D\r\n      1662  1FFFFFFF   00000004    8        00\t20\tFF\tFF\tFF\tFF\tFF\tFF\r\n      1652  1FFFFFFF   00000004    8        00\t20\tFF\tFF\tFF\tFF\tFF\tFF\r\n      1649  1FFFFFFF   00000004    8        00\t00\tFF\tFF\tFF\tFF\tFF\tFF\r\n      1649  18FEF117   00000004    8        F7\t97\tCC\tCF\tFF\tFF\tFF\tFF\r\n      1648  18FB01A7   00000004    8        FF\t1F\tFF\tFF\tFF\tFF\tFF\tFF\r\n      1648  18F121F0   00000004    8        09\t18\t00\t00\tFF\tFF\tB0\t01\r\n      1683  0CF102A7   00000004    8        30\t75\tE0\t2E\t80\tFF\tFF\tFD\r\n      1683  0CF101A7   00000004    8        68\t00\t97\tCC\t00\t16\t39\t6E\r\n      1682  1FFFFFFF   00000004    8        00\t00\tFF\tFF\tFF\tFF\tFF\tFF\r\n      1672  1FFFFFFF   00000004    8        00\t00\tFF\tFF\tFF\tFF\tFF\tFF\r\n      1663  0CF102A7   00000004    8        30\t75\tE0\t2E\t80\tFF\tFF\tFD\r\n      1663  0CF101A7   00000004    8        68\t00\t97\tCC\t00\t16\t39\t6D\r\n      1662  1FFFFFFF   00000004    8        00\t20\tFF\tFF\tFF\tFF\tFF\tFF\r\n      1652  1FFFFFFF   00000004    8        00\t20\tFF\tFF\tFF\tFF\tFF\tFF\r\n      1649  1FFFFFFF   00000004    8        00\t00\tFF\tFF\tFF\tFF\tFF\tFF\r\n      1649  18FEF117   00000004    8        F7\t97\tCC\tCF\tFF\tFF\tFF\tFF\r\n      1648  18FB01A7   00000004    8        FF\t1F\tFF\tFF\tFF\tFF\tFF\tFF\r\n      1692  1FFFFFFF   00000004    8        00\t20\tFF\tFF\tFF\tFF\tFF\tFF\r\n      1683  0CF102A7   00000004    8        30\t75\tE0\t2E\t80\tFF\tFF\tFD\r\n      1683  0CF101A7   00000004    8        68\t00\t97\tCC\t00\t16\t39\t6E\r\n      1682  1FFFFFFF   00000004    8        00\t00\tFF\tFF\tFF\tFF\tFF\tFF\r\n      1672  1FFFFFFF   00000004    8        00\t00\tFF\tFF\tFF\tFF\tFF\tFF\r\n      1663  0CF102A7   00000004    8        30\t75\tE0\t2E\t80\tFF\tFF\tFD\r\n      1663  0CF101A7   00000004    8        68\t00\t97\tCC\t00\t16\t39\t6D\r\n      1662  1FFFFFFF   00000004    8        00\t20\tFF\tFF\tFF\tFF\tFF\tFF\r\n      1652  1FFFFFFF   00000004    8        00\t20\tFF\tFF\tFF\tFF\tFF\tFF\r\n      1649  1FFFFFFF   00000004    8        00\t00\tFF\tFF\tFF\tFF\tFF\tFF\r\n      1649  18FEF117   00000004    8        F7\t97\tCC\tCF\tFF\tFF\tFF\tFF\r\n      1693  18F106A7   00000004    8        00\tF7\tFF\tFF\tFF\tFF\tFF\t92\r\n      1692  1FFFFFFF   00000004    8        00\t20\tFF\tFF\tFF\tFF\tFF\tFF\r\n      1683  0CF102A7   00000004    8        30\t75\tE0\t2E\t80\tFF\tFF\tFD\r\n      1683  0CF101A7   00000004    8        68\t00\t97\tCC\t00\t16\t39\t6E\r\n      1682  1FFFFFFF   00000004    8        00\t00\tFF\tFF\tFF\tFF\tFF\tFF\r\n      1672  1FFFFFFF   00000004    8        00\t00\tFF\tFF\tFF\tFF\tFF\tFF\r\n      1663  0CF102A7   00000004    8        30\t75\tE0\t2E\t80\tFF\tFF\tFD\r\n      1663  0CF101A7   00000004    8        68\t00\t97\tCC\t00\t16\t39\t6D\r\n      1662  1FFFFFFF   00000004    8        00\t20\tFF\tFF\tFF\tFF\tFF\tFF\r\n      1652  1FFFFFFF   00000004    8        00\t20\tFF\tFF\tFF\tFF\tFF\tFF\r\n      1649  1FFFFFFF   00000004    8        00\t00\tFF\tFF\tFF\tFF\tFF\tFF\r\n      1702  1FFFFFFF   00000004    8        00\t00\tFF\tFF\tFF\tFF\tFF\tFF\r\n      1693  18F106A7   00000004    8        00\tF7\tFF\tFF\tFF\tFF\tFF\t92\r\n      1692  1FFFFFFF   00000004    8        00\t20\tFF\tFF\tFF\tFF\tFF\tFF\r\n      1683  0CF102A7   00000004    8        30\t75\tE0\t2E\t80\tFF\tFF\tFD\r\n      1683  0CF101A7   00000004    8        68\t00\t97\tCC\t00\t16\t39\t6E\r\n      1682  1FFFFFFF   00000004    8        00\t00\tFF\tFF\tFF\tFF\tFF\tFF\r\n      1672  1FFFFFFF   00000004    8        00\t00\tFF\tFF\tFF\tFF\tFF\tFF\r\n      1663  0CF102A7   00000004    8        30\t75\tE0\t2E\t80\tFF\tFF\tFD\r\n      1663  0CF101A7   00000004    8        68\t00\t97\tCC\t00\t16\t39\t6D\r\n      1662  1FFFFFFF   00000004    8        00\t20\tFF\tFF\tFF\tFF\tFF\tFF\r\n      1652  1FFFFFFF   00000004    8        00\t20\tFF\tFF\tFF\tFF\tFF\tFF\r\n      1703  0CF101A7   00000004    8        68\t00\t97\tCC\t00\t16\t39\t6F\r\n      1702  1FFFFFFF   00000004    8        00\t00\tFF\tFF\tFF\tFF\tFF\tFF\r\n      1693  18F106A7   00000004    8        00\tF7\tFF\tFF\tFF\tFF\tFF\t92\r\n      1692  1FFFFFFF   00000004    8        00\t20\tFF\tFF\tFF\tFF\tFF\tFF\r\n      1683  0CF102A7   00000004    8        30\t75\tE0\t2E\t80\tFF\tFF\tFD\r\n      1683  0CF101A7   00000004    8        68\t00\t97\tCC\t00\t16\t39\t6E\r\n      1682  1FFFFFFF   00000004    8        00\t00\tFF\tFF\tFF\tFF\tFF\tFF\r\n      1672  1FFFFFFF   00000004    8        00\t00\tFF\tFF\tFF\tFF\tFF\tFF\r\n      1663  0CF102A7   00000004    8        30\t75\tE0\t2E\t80\tFF\tFF\tFD\r\n      1663  0CF101A7   00000004    8        68\t00\t97\tCC\t00\t16\t39\t6D\r\n      1662  1FFFFFFF   00000004    8        00\t20\tFF\tFF\tFF\tFF\tFF\tFF\r\n      1703  0CF102A7   00000004    8        30\t75\tE0\t2E\t80\tFF\tFF\tFD\r\n      1703  0CF101A7   00000004    8        68\t00\t97\tCC\t00\t16\t39\t6F\r\n      1702  1FFFFFFF   00000004    8        00\t00\tFF\tFF\tFF\tFF\tFF\tFF\r\n      1693  18F106A7   00000004    8        00\tF7\tFF\tFF\tFF\tFF\tFF\t92\r\n      1692  1FFFFFFF   00000004    8        00\t20\tFF\tFF\tFF\tFF\tFF\tFF\r\n      1683  0CF102A7   00000004    8        30\t75\tE0\t2E\t80\tFF\tFF\tFD\r\n      1683  0CF101A7   00000004    8        68\t00\t97\tCC\t00\t16\t39\t6E\r\n      1682  1FFFFFFF   00000004    8        00\t00\tFF\tFF\tFF\tFF\tFF\tFF\r\n      1672  1FFFFFFF   00000004    8        00\t00\tFF\tFF\tFF\tFF\tFF\tFF\r\n      1663  0CF102A7   00000004    8        30\t75\tE0\t2E\t80\tFF\tFF\tFD\r\n      1663  0CF101A7   00000004    8        68\t00\t97\tCC\t00\t16\t39\t6D\r\n      1712  1FFFFFFF   00000004    8        00\t20\tFF\tFF\tFF\tFF\tFF\tFF\r\n      1703  0CF102A7   00000004    8        30\t75\tE0\t2E\t80\tFF\tFF\tFD\r\n      1703  0CF101A7   00000004    8        68\t00\t97\tCC\t00\t16\t39\t6F\r\n      1702  1FFFFFFF   00000004    8        00\t00\tFF\tFF\tFF\tFF\tFF\tFF\r\n      1693  18F106A7   00000004    8        00\tF7\tFF\tFF\tFF\tFF\tFF\t92\r\n      1692  1FFFFFFF   00000004    8        00\t20\tFF\tFF\tFF\tFF\tFF\tFF\r\n      1683  0CF102A7   00000004    8        30\t75\tE0\t2E\t80\tFF\tFF\tFD\r\n      1683  0CF101A7   00000004    8        68\t00\t97\tCC\t00\t16\t39\t6E\r\n      1682  1FFFFFFF   00000004    8        00\t00\tFF\tFF\tFF\tFF\tFF\tFF\r\n      1672  1FFFFFFF   00000004    8        00\t00\tFF\tFF\tFF\tFF\tFF\tFF\r\n      1663  0CF102A7   00000004    8        30\t75\tE0\t2E\t80\tFF\tFF\tFD\r\n      1722  1FFFFFFF   00000004    8        00\t20\tFF\tFF\tFF\tFF\tFF\tFF\r\n      1712  1FFFFFFF   00000004    8        00\t20\tFF\tFF\tFF\tFF\tFF\tFF\r\n      1703  0CF102A7   00000004    8        30\t75\tE0\t2E\t80\tFF\tFF\tFD\r\n      1703  0CF101A7   00000004    8        68\t00\t97\tCC\t00\t16\t39\t6F\r\n      1702  1FFFFFFF   00000004    8        00\t00\tFF\tFF\tFF\tFF\tFF\tFF\r\n      1693  18F106A7   00000004    8        00\tF7\tFF\tFF\tFF\tFF\tFF\t92\r\n      1692  1FFFFFFF   00000004    8        00\t20\tFF\tFF\tFF\tFF\tFF\tFF\r\n      1683  0CF102A7   00000004    8        30\t75\tE0\t2E\t80\tFF\tFF\tFD\r\n      1683  0CF101A7   00000004    8        68\t00\t97\tCC\t00\t16\t39\t6E\r\n      1682  1FFFFFFF   00000004    8        00\t00\tFF\tFF\tFF\tFF\tFF\tFF\r\n      1672  1FFFFFFF   00000004    8        00\t00\tFF\tFF\tFF\tFF\tFF\tFF\r\n      1723  0CF101A7   00000004    8        68\t00\t97\tCC\t00\t16\t39\t70\r\n      1722  1FFFFFFF   00000004    8        00\t20\tFF\tFF\tFF\tFF\tFF\tFF\r\n      1712  1FFFFFFF   00000004    8        00\t20\tFF\tFF\tFF\tFF\tFF\tFF\r\n      1703  0CF102A7   00000004    8        30\t75\tE0\t2E\t80\tFF\tFF\tFD\r\n      1703  0CF101A7   00000004    8        68\t00\t97\tCC\t00\t16\t39\t6F\r\n      1702  1FFFFFFF   00000004    8        00\t00\tFF\tFF\tFF\tFF\tFF\tFF\r\n      1693  18F106A7   00000004    8        00\tF7\tFF\tFF\tFF\tFF\tFF\t92\r\n      1692  1FFFFFFF   00000004    8        00\t20\tFF\tFF\tFF\tFF\tFF\tFF\r\n      1683  0CF102A7   00000004    8        30\t75\tE0\t2E\t80\tFF\tFF\tFD\r\n      1683  0CF101A7   00000004    8        68\t00\t97\tCC\t00\t16\t39\t6E\r\n      1682  1FFFFFFF   00000004    8        00\t00\tFF\tFF\tFF\tFF\tFF\tFF\r\n      1723  0CF102A7   00000004    8        30\t75\tE0\t2E\t80\tFF\tFF\tFD\r\n      1723  0CF101A7   00000004    8        68\t00\t97\tCC\t00\t16\t39\t70\r\n      1722  1FFFFFFF   00000004    8        00\t20\tFF\tFF\tFF\tFF\tFF\tFF\r\n      1712  1FFFFFFF   00000004    8        00\t20\tFF\tFF\tFF\tFF\tFF\tFF\r\n      1703  0CF102A7   00000004    8        30\t75\tE0\t2E\t80\tFF\tFF\tFD\r\n      1703  0CF101A7   00000004    
